vi "ex14-5(subVI).vi"(1 "輸入":dbl) -> (0 "溢位?65536":bool)   [LabVIEW 2014]
uses:
  <vilib>/NXT/Subs/MotorOutput.ctl
  <vilib>/NXT/Dual Mode Library/prims/inRangeAndCoerce/inRangeAndCoerce_float.vi
  <vilib>/NXT/Dual Mode Library/Motors/MotorDistance_Single.vi
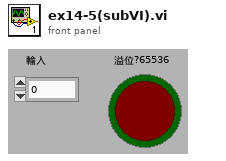
[diagram p1: front panel]
types:
  T1 = typedef "MotorOutput.ctl" = u8
  T2 = typedef "LVHSConnector.ctl" = refnum<class "BrickReference.lvclass">
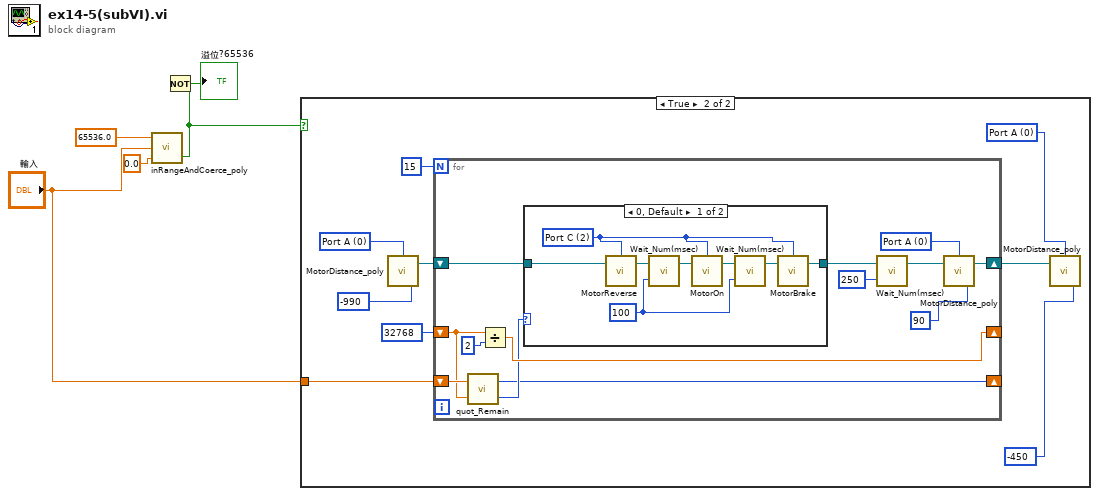
[diagram p0: block diagram]
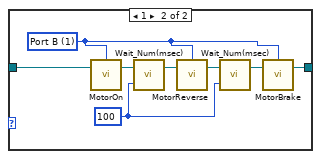
[diagram p3: hidden frame]
diagram:
  n1 = call-poly <vilib>:"inRangeAndCoerce_poly.vi"("lower limit"=0.0, "x"="輸入", "upper limit"=65536.0 ("y")) -> ("In Range?"=w4:bool)  [unwired: 1 out]
  n2 = Not(x=w4) -> (.not. x?=→"溢位?65536":bool)
  n3 = case shown="True" w4 {
    tunnel: "輸入" -> [_ w13]
    frame False {
    }
    frame True {
      w6 = T1 0 items=["Port A", "Port B", "Port C", "All Ports"] ("Output Port (All Ports)")
      w7 = T1 0 items=["Port A", "Port B", "Port C", "All Ports"] ("Output Port (All Ports)")
      n4 = call-poly <vilib>:"MotorDistance_poly.vi"("Angle of Rotation (360)"=-990 ("Distance (100)"), "Output Port (All Ports)"=w7) -> ("NXT/EV3"=w11:T2)  [unwired: 2 in]
      n5 = for {
        N: 15 -> [_]
        shift-right: [w15] -> _
        shift-left: w13 -> [w19]
        shift-right: [w26] -> _
        shift-left: 32768 -> [w18]
        shift-right: [w23] -> w10
        shift-left: w11 -> [w25]
        w16 = T1 0 items=["Port A", "Port B", "Port C", "All Ports"] ("Output Port (All Ports)")
        n6 = call <vilib>:"quot_Remain.vi"("y"=w18, "x"=w19) -> ("floor(x/y)"=w17:i32, "x-y*floor(x/y)"=w15:i32)
        n7 = Divide(x=w18, y=2) -> (x/y=w26:dbl)
        n8 = case shown="0, Default" w17 {
          tunnel: w25 -> [w31 w38]
          tunnel: [w32 w37] -> w22
          frame 0, Default {
            w33 = u32 100 ("Time (100 msec)")
            w35 = T1 2 items=["Port A", "Port B", "Port C", "All Ports"] ("Output Port (All Ports)")
            n9 = call <vilib>:"MotorReverse.vi"("NXT/EV3"=w31, "Output Port (All Ports)"=w35) -> ("NXT/EV3"=w30:T2)  [unwired: 2 in]
            n10 = call <vilib>:"Wait_Num(msec).vi"("Time (100 msec)"=w33, "NXT/EV3"=w30) -> ("NXT/EV3"=w29:T2)  [unwired: 2 in]
            n11 = call <vilib>:"MotorOn.vi"("NXT/EV3"=w29, "Output Port (All Ports)"=w35) -> ("NXT/EV3"=w28:T2)  [unwired: 2 in]
            n12 = call <vilib>:"Wait_Num(msec).vi"("Time (100 msec)"=w33, "NXT/EV3"=w28) -> ("NXT/EV3"=w34:T2)  [unwired: 2 in]
            n13 = call <vilib>:"MotorBrake.vi"("NXT/EV3"=w34, "Port (All Ports)"=w35) -> ("NXT/EV3"=w32:T2)  [unwired: 2 in]
          }
          frame 1 {
            w36 = u32 100 ("Time (100 msec)")
            w43 = T1 1 items=["Port A", "Port B", "Port C", "All Ports"] ("Output Port (All Ports)")
            n14 = call <vilib>:"MotorOn.vi"("NXT/EV3"=w38, "Output Port (All Ports)"=w43) -> ("NXT/EV3"=w39:T2)  [unwired: 2 in]
            n15 = call <vilib>:"Wait_Num(msec).vi"("Time (100 msec)"=w36, "NXT/EV3"=w39) -> ("NXT/EV3"=w40:T2)  [unwired: 2 in]
            n16 = call <vilib>:"MotorReverse.vi"("NXT/EV3"=w40, "Output Port (All Ports)"=w43) -> ("NXT/EV3"=w41:T2)  [unwired: 2 in]
            n17 = call <vilib>:"Wait_Num(msec).vi"("Time (100 msec)"=w36, "NXT/EV3"=w41) -> ("NXT/EV3"=w42:T2)  [unwired: 2 in]
            n18 = call <vilib>:"MotorBrake.vi"("NXT/EV3"=w42, "Port (All Ports)"=w43) -> ("NXT/EV3"=w37:T2)  [unwired: 2 in]
          }
        }
        n19 = call <vilib>:"Wait_Num(msec).vi"("Time (100 msec)"=u32 250, "NXT/EV3"=w22) -> ("NXT/EV3"=w21:T2)  [unwired: 2 in]
        n20 = call-poly <vilib>:"MotorDistance_poly.vi"("Angle of Rotation (360)"=90 ("Distance (100)"), "NXT/EV3"=w21, "Output Port (All Ports)"=w16) -> ("NXT/EV3"=w23:T2)  [unwired: 1 in]
      }
      n21 = call-poly <vilib>:"MotorDistance_poly.vi"("Angle of Rotation (360)"=-450 ("Distance (100)"), "NXT/EV3"=w10, "Output Port (All Ports)"=w6) -> ()  [unwired: 1 in, 1 out]
    }
  }
